vi "S2C_ExeScriptIncRow.vi"(8 "Error In":errorcluster) -> (0 "Error Out":errorcluster)   [LabVIEW 2015]
doc: "Determines the top row to display for auto-scrolling, and checks for the presents of a breakpoint."
uses:
  Globals/S2C_Globals.vi
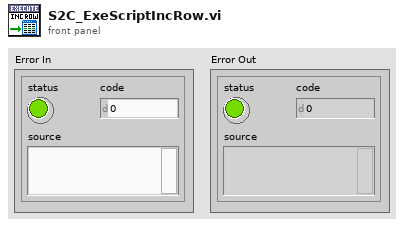
[diagram p1: front panel]
types:
  T1 = typedef "LVRowAndColumnUnsignedTypeDef.ctl" = cluster{"Row":u32, "Column":u32}
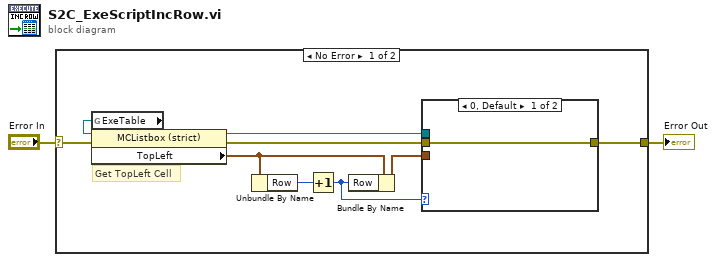
[diagram p0: block diagram]
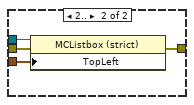
[diagram p2: hidden frame]
diagram:
  n1 = case shown="No Error" "Error In" {
    selector: "Error In" -> [w11 w17]
    tunnel: [w3 w17] -> w1
    frame No Error {
      # "Get TopLeft Cell"
      n2 = global read "S2C_Globals.vi" "ExeTable"() -> (w10:refnum<vi>)
      n3 = property class="MCListbox (strict)"(reference=w10, error in=w11) -> (reference out=w4:refnum<vi>, error out=w7:errorcluster, "TopLeft"=w9:T1)
      n4 = Unbundle By Name(w9) -> ("Row"=w8:u32)
      n5 = Increment(x=w8) -> (x+1=w6:u32)
      n6 = Bundle By Name(cluster=w9, "Row"=w6) -> (w5:T1)
      n7 = case shown="0, Default" w6 {
        tunnel: w7 -> [w12 w16]
        tunnel: w5 -> [_ w15]
        tunnel: w4 -> [_ w14]
        tunnel: [w12 w13] -> w3
        frame 0, Default {
        }
        frame 2.. {
          n8 = property class="MCListbox (strict)"(reference=w14, error in=w16, "TopLeft"=w15) -> (error out=w13:errorcluster)  [unwired: 1 out]
        }
      }
    }
    frame Error {
    }
  }
  "Error Out" <- w1
